vi "Scale Color OLD.vi"(4 "Brightness":u8, 6 "Factor":dbl, 9 "Red":u8, 10 "Green":u8, 11 "Blue":u8) -> (1 "Red Out":u8, 2 "Green Out":u8, 3 "Blue Out":u8)   [LabVIEW 2013]
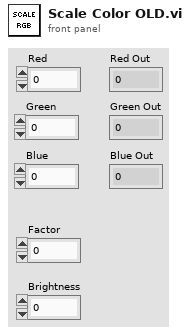
[diagram p1: front panel]
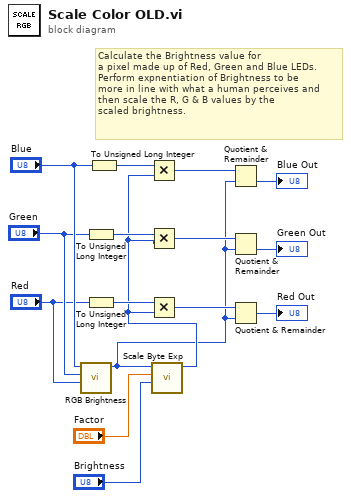
[diagram p0: block diagram]
diagram:
  # "Calculate the Brightness value for\na pixel made up of Red, Green and Blue LEDs.\nPerform expnentiation of Brightness to be\nmore in line with what a human perceives and\nthen scale the R, G & B values by the \nscaled brightness."
  n1 = call "RGB Brightness.vi"("Red"="Red", "Green"="Green", "Blue"="Blue") -> ("Brightness"=w1:u8)  [unwired: 8 in]
  n2 = To Unsigned Long Integer(number="Green") -> (unsigned 32bit integer=w5:u32)
  n3 = To Unsigned Long Integer(number="Red") -> (unsigned 32bit integer=w3:u32)
  n4 = To Unsigned Long Integer(number="Blue") -> (unsigned 32bit integer=w7:u32)
  n5 = call "Scale Byte Exp.vi"("Brightness"="Brightness", "Factor"="Factor", "Byte"=w1) -> ("Byte Scaled"=w2:u8)  [unwired: 8 in]
  n6 = Multiply(x=w7, y=w2) -> (x*y=w14:u32)
  n7 = Multiply(x=w5, y=w2) -> (x*y=w12:u32)
  n8 = Multiply(x=w3, y=w2) -> (x*y=w10:u32)
  n9 = Quotient & Remainder(x=w14, y=w1) -> (floor(x/y)=→"Blue Out":u32)  [unwired: 1 out]
  n10 = Quotient & Remainder(x=w12, y=w1) -> (floor(x/y)=→"Green Out":u32)  [unwired: 1 out]
  n11 = Quotient & Remainder(x=w10, y=w1) -> (floor(x/y)=→"Red Out":u32)  [unwired: 1 out]
